vi "Monochromator Wavelength to Colour Wheel Enum.vi"(8 "error in (no error)":errorcluster, 10 "Possible Wavelengths":dbl[](array[numeric])=[0.0, 435.0, 590.0, 665.0, 715.0, 850.0, 1000.0], 11 "Wavelength (nm)":dbl=500.0 format="%#_13g") -> (0 "error out":errorcluster, 3 "Index":i32)   [LabVIEW 2017, in "Colour Wheel.lvlib"]
uses:
  Colour Wheel.lvlib
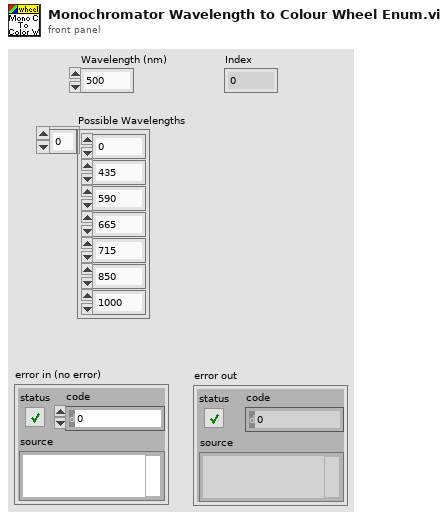
[diagram p1: front panel]
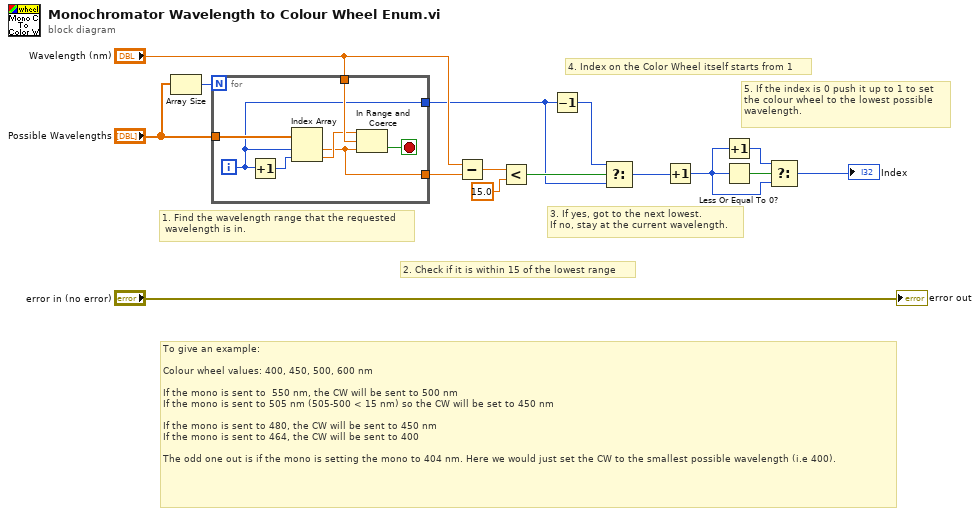
[diagram p0: block diagram]
diagram:
  # "3. If yes, got to the next lowest.\nIf no, stay at the current wavelength."
  # "2. Check if it is within 15 of the lowest range"
  # "1. Find the wavelength range that the requested\n wavelength is in."
  # "To give an example:\n\nColour wheel values: 400, 450, 500, 600 nm\n\nIf the mono is sent to  550 nm, the CW will be sent to 500 nm\nIf the mono is sent to 505 nm (505-500 < 15 nm) so the CW will be set to 450 nm\n\nIf the mono is sent to 480, the CW will be sent to 450 nm\nIf the mono is sent to 464, the CW will be sent to 400\n\nThe odd one out is if the mono is setting the mono to 404 nm. Here we would just set the CW to the smallest possible wavelength (i.e 400)."
  # "5. If the index is 0 push it up to 1 to set\nthe colour wheel to the lowest possible\nwavelength."
  # "4. Index on the Color Wheel itself starts from 1"
  n1 = Array Size(array="Possible Wavelengths") -> (size(s)=w5:i32)
  n2 = for {
    N: w5 -> [_]
    tunnel: "Possible Wavelengths" -> [w22]
    tunnel: "Wavelength (nm)" -> [w20]
    tunnel: [w17] -> w6
    tunnel: [w16] -> w11
    i -> [w17]
    stop <- w18 stop-if-true
    n3 = Increment(x=w17) -> (x+1=w21:i32)
    n4 = Index Array(array=w22, index #1=w17, index #2=w21) -> (element #1=w16:dbl, element #2=w19:dbl)
    n5 = In Range and Coerce(upper limit=w19, x=w20, lower limit=w16) -> (In Range?=w18:bool)  [unwired: 1 out]
  }
  n6 = Subtract(x="Wavelength (nm)", y=w11) -> (x-y=w10:dbl)
  n7 = Less?(x=w10, y=15.0) -> (x < y?=w8:bool)
  n8 = Decrement(x=w6) -> (x-1=w7:i32)
  n9 = Select(t=w7, s=w8, f=w6) -> (s? t:f=w12:i32)
  n10 = Increment(x=w12) -> (x+1=w3:i32)
  n11 = Increment(x=w3) -> (x+1=w1:i32)
  n12 = Less Or Equal To 0?(x=w3) -> (x <= 0?=w2:bool)
  n13 = Select(t=w1, s=w2, f=w3) -> (s? t:f=→"Index":i32)
  "error out" <- "error in (no error)"
